vi "AprilTagPoseEstimator_New.vi"(7 "TagSize_m":dbl, 8 "Cy_pix":dbl, 9 "Cx_pix":dbl, 10 "Fy_pix":dbl, 11 "Fx_pix":dbl) -> (3 "AprilTagPoseEstimator":T1)   [LabVIEW 2019, in "Trajectory_Library.lvlib"]
uses:
  Trajectory_Library.lvlib
  TypeDef/APRIL_TAG_POSE_ESTIMATOR.ctl
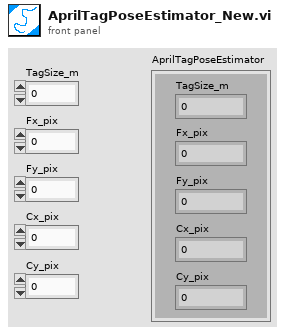
[diagram p1: front panel]
types:
  T1 = typedef "Trajectory_Library.lvlib/APRIL_TAG_POSE_ESTIMATOR.ctl" = cluster{"TagSize_m":dbl, "Fx_pix":dbl, "Fy_pix":dbl, "Cx_pix":dbl, "Cy_pix":dbl}
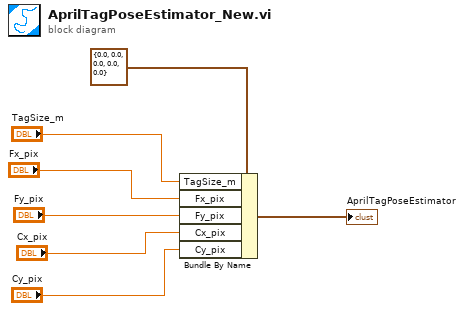
[diagram p0: block diagram]
diagram:
  n1 = Bundle By Name(cluster=T1 {"TagSize_m"=0.0, "Fx_pix"=0.0, "Fy_pix"=0.0, "Cx_pix"=0.0, "Cy_pix"=0.0} ("AprilTagPoseEstimator"), "TagSize_m"="TagSize_m", "Fx_pix"="Fx_pix", "Fy_pix"="Fy_pix", "Cx_pix"="Cx_pix", "Cy_pix"="Cy_pix") -> (→"AprilTagPoseEstimator":T1)
